vi "SetI.vi"(8 "error in (no error)":errorcluster, 10 "i":i32, 11 "reference in":refnum<class "GOOP4_Base.lvclass">) -> (0 "error out":errorcluster, 3 "reference out":refnum<class "GOOP4_Base.lvclass">)   [LabVIEW 2019, in "GOOP4_Base.lvclass"]
uses:
  GOOP4_Base.lvclass
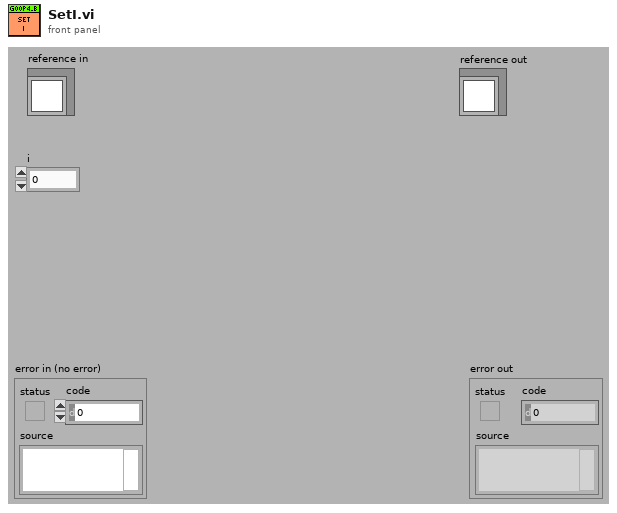
[diagram p1: front panel]
types:
  T1 = typedef "GOOP4_Base.lvclass/ObjectAttributes.ctl" = cluster{"i":i32}
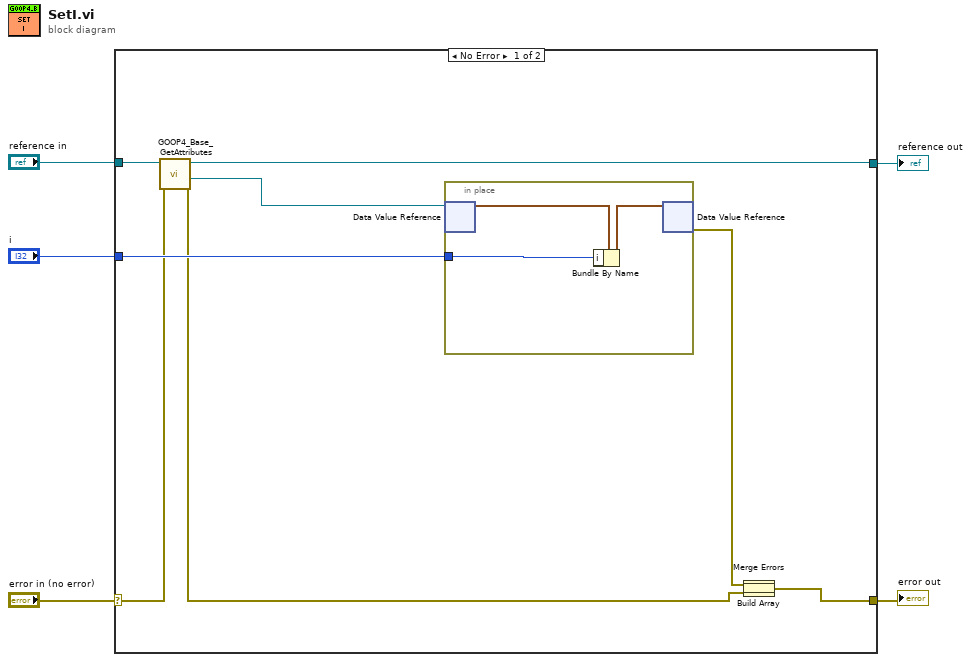
[diagram p0: block diagram]
diagram:
  n1 = case shown="No Error" "error in (no error)" {
    selector: "error in (no error)" -> [w8 w19]
    tunnel: [w12 w19] -> w4
    tunnel: [w10 w18] -> w2
    tunnel: "reference in" -> [w11 w18]
    tunnel: "i" -> [w14 _]
    frame No Error {
      n2 = call "GOOP4_Base_GetAttributes.vi"("error in (no error)"=w8, "reference in"=w11) -> ("error out"=w7:errorcluster, "DataRef"=w9:refnum<data-value>, "reference out"=w10:refnum<class "GOOP4_Base.lvclass">)  [unwired: 6 in, 1 out]
      n3 = in-place {
        in-place-border: w14 -> [w17]
        n4 = in-place-dvr #1(w9) -> (w16:T1)  [unwired: 1 out]
        n5 = Bundle By Name(cluster=w16, "i"=w17) -> (w15:T1)
        n6 = in-place-dvr #1(w15) -> (w13:errorcluster)  [unwired: 1 out]
      }
      n7 = Build Array(w13, w7) -> (w6:errorcluster[])
      n8 = Merge Errors(w6) -> (w12:errorcluster)
    }
    frame Error {
    }
  }
  "error out" <- w4
  "reference out" <- w2
